vi "concatenate_wavetext.vi"(0 "Specimen":string, 1 "Date":string, 2 "Time":string, 5 "Temp":string, 7 "Species":string, 9 "Coupling":string, 12 "Location":string, 13 "Gain":string, 14 "Comments":string) -> (11 "concatenated string":string)   [LabVIEW 2014]
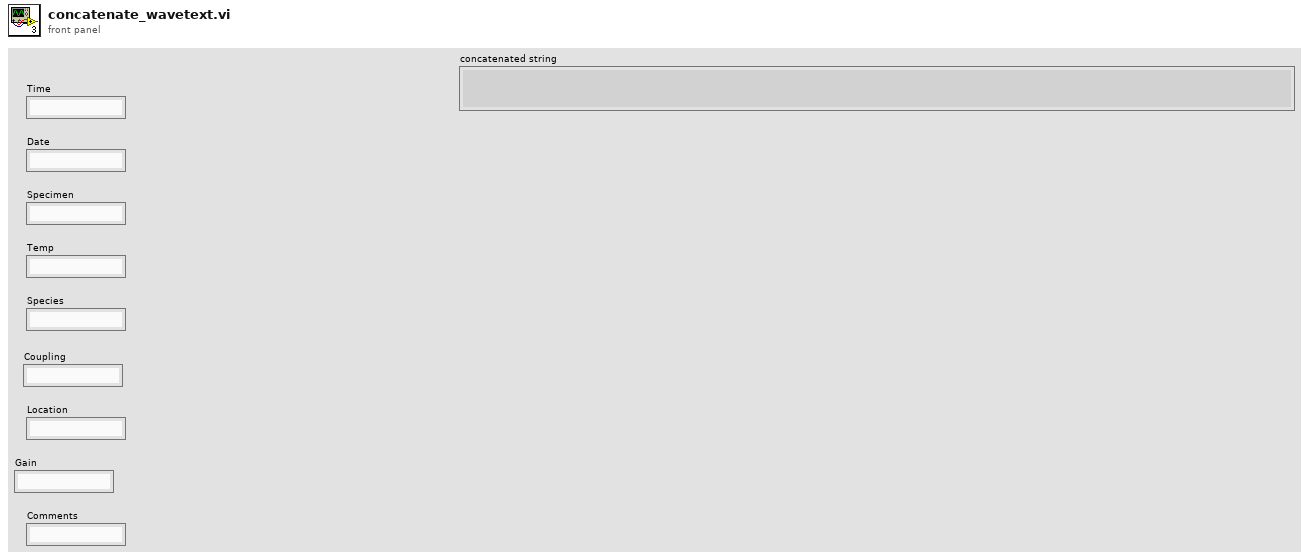
[diagram p1: front panel]
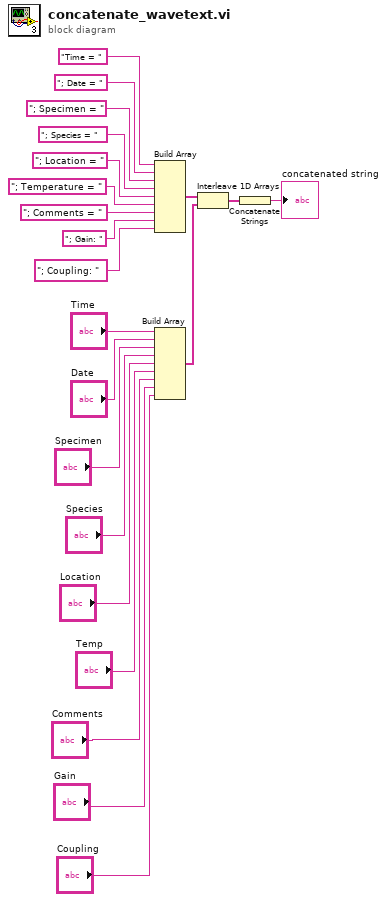
[diagram p0: block diagram]
diagram:
  n1 = Build Array("Time = ", "; Date = ", "; Specimen = ", "; Species = ", "; Location = ", "; Temperature = ", "; Comments = ", "; Gain: ", "; Coupling: ") -> (w21:string[])
  n2 = Build Array("Time", "Date", "Specimen", "Species", "Location", "Temp", "Comments", "Gain", "Coupling") -> (w22:string[])
  n3 = Interleave 1D Arrays(w21, w22) -> (w5:string[])
  n4 = Concatenate Strings(w5) -> (→"concatenated string":string)
